vi "Get Contact.vi"(8 "error in (no error)":errorcluster, 11 "UUID":string) -> (0 "error out":errorcluster, 2 "Contact":T1, 3 "UUID dup":string)   [LabVIEW 2014, in "Map Data.lvlib"]
doc: "Retrieves a single contact by ID from the address book data store."
uses:
  Map Data.lvlib
  MapCommand.ctl
  MapDatas.ctl
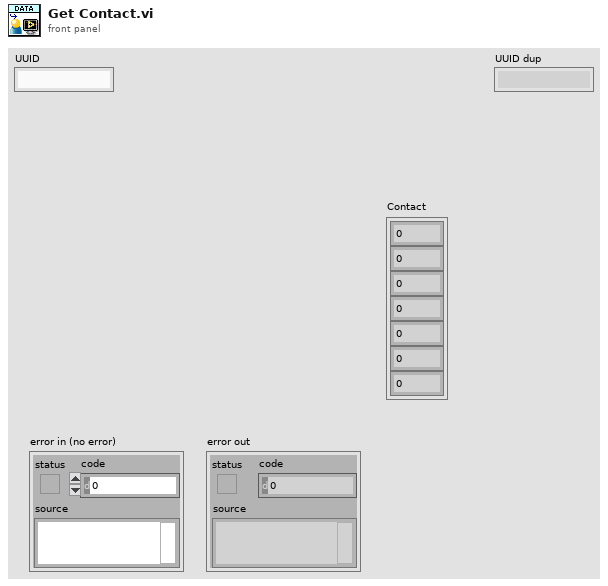
[diagram p1: front panel]
types:
  T1 = typedef "Map Data.lvlib/MapDatas.ctl" = cluster{"X":dbl, "Y":dbl, "Z":dbl, "heading":dbl, "X2":dbl, "Y2":dbl, "Z2":dbl}
  T2 = typedef "Map Data.lvlib/MapCommand.ctl" = enum16{"Load", "Update Cursor", "Save", "Get All Data", "Get Single Data", "Set Single Data", "Delete All", "Remove Single Data", "Set Favorite Status", "Is Data Modified", "Import Data"}
  T3 = typedef "Map Data.lvlib/All-Lines.ctl" = T4[]
  T4 = typedef "Map Data.lvlib/LineCluster.ctl" = cluster{"Line name":string, "Line array":cluster{"X":dbl, "Y":dbl, "Z":dbl}[], "Line connections":T5[]}
  T5 = typedef "LineConnection.ctl" = cluster{"Index":i32, "Switch Pos":cluster{"X":dbl, "Y":dbl, "Z":dbl}, "Switch operational":bool, "Switch State":bool, "Connection Index":i32, "Connection Pos":cluster{"X":dbl, "Y":dbl, "Z":dbl}, "LinePos Index":i32, "ConnectPos Index":i32, "Same direction?":bool, "Manual Overide":bool, "Manual State":bool}
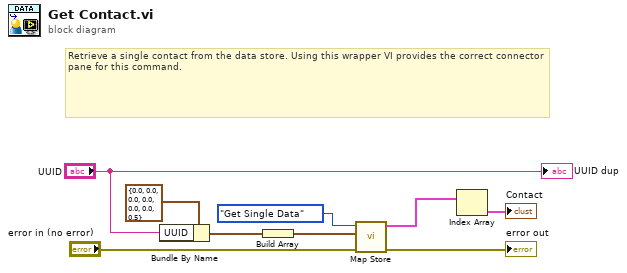
[diagram p0: block diagram]
diagram:
  # "Retrieve a single contact from the data store. Using this wrapper VI provides the correct connector pane for this command."
  n1 = Bundle By Name(cluster=T1 {"X"=0.0, "Y"=0.0, "Z"=0.0, "heading"=0.0, "X2"=0.0, "Y2"=0.0, "Z2"=0.5} ("Contact"), "UUID"="UUID") -> (w8:T1)
  n2 = Build Array(w8) -> (w3:T1[])
  n3 = call "Map Store.vi"("error in (no error)"="error in (no error)", "All Lines"=w3, "Command"=MapCommand."Get Single Data") -> ("error out"=→"error out":errorcluster, "All Lines out"=w4:T3)  [unwired: 5 in, 2 out]
  n4 = Index Array(array=w4) -> (element=→"Contact":T4)  [unwired: 1 in]
  "UUID dup" <- "UUID"
